vi "Set Temperature.vi"(8 "error in (no error)":errorcluster, 10 "Setpoint":dbl, 11 "HotCoil Settings":T1) -> (0 "error out":errorcluster, 1 "Connection Error":bool, 3 "HotCoil Settings":T1)   [LabVIEW 2021, in "HotCoil.lvlib"]
uses:
  HotCoil.lvlib
  HotCoil Settings.ctl
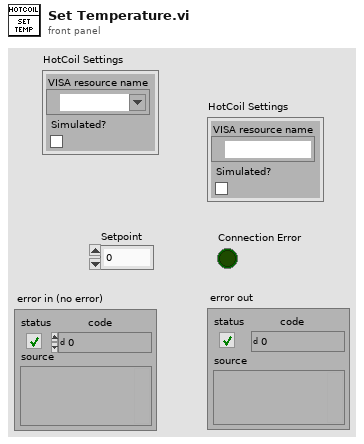
[diagram p1: front panel]
types:
  T1 = typedef "HotCoil.lvlib/HotCoil Settings.ctl" = cluster{"VISA resource name":refnum<visa-resource-name>, "Simulated?":bool}
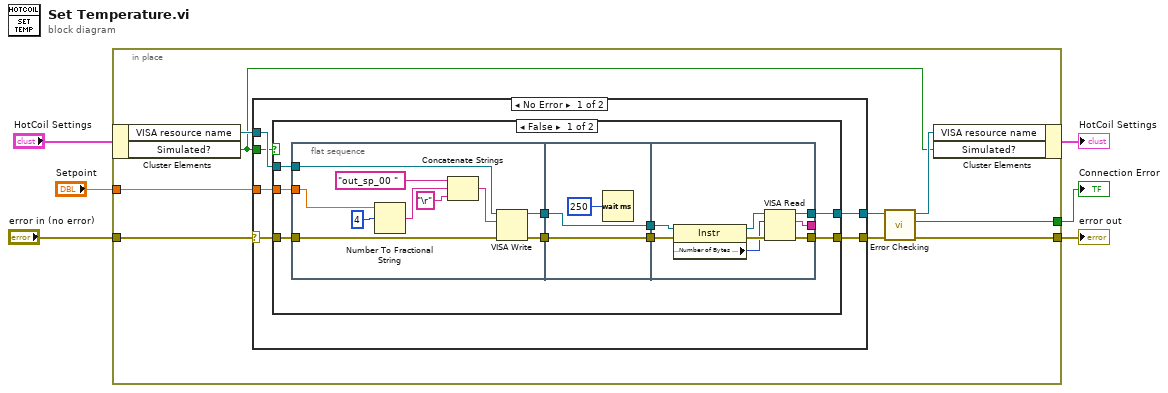
[diagram p0: block diagram]
diagram:
  n1 = in-place {
    in-place-border: "error in (no error)" -> [w15]
    in-place-border: [w12] -> w5
    in-place-border: [w11] -> w4
    in-place-border: "Setpoint" -> [w8]
    n2 = in-place-cluster #1("HotCoil Settings") -> ("VISA resource name"=w10:refnum<visa-resource-name>, "Simulated?"=w7:bool)
    n3 = case shown="No Error" w15 {
      selector: w15 -> [w21 w55]
      tunnel: [w20 w55] -> w13
      tunnel: [w19 w54] -> w14
      tunnel: w10 -> [w18 w54]
      tunnel: w8 -> [w17 _]
      tunnel: w7 -> [w16 _]
      frame No Error {
        n4 = case shown="False" w16 {
          tunnel: w21 -> [w25 w53]
          tunnel: [w23 w53] -> w20
          tunnel: [w24 w52] -> w19
          tunnel: w18 -> [w26 w52]
          tunnel: w17 -> [w22 _]
          frame False {
            n5 = flat-sequence {
              tunnel: w25 -> [w40]
              tunnel: w26 -> [w39]
              tunnel: [w38] -> w30
              tunnel: [w37] -> w29
              tunnel: w22 -> [w36]
              tunnel: w30 -> [w43]
              tunnel: [w43] -> w28
              tunnel: w29 -> [w42]
              tunnel: [w42] -> w27
              tunnel: [w51] -> w23
              tunnel: [w50] -> _
              tunnel: [w49] -> w24
              tunnel: w28 -> [w48]
              tunnel: w27 -> [w47]
              frame #0 {
                n6 = Number To Fractional String(number=w36, width (-)=i16 4) -> (F-format string=w33:string)  [unwired: 2 in]
                n7 = Concatenate Strings("out_sp_00 " ("write buffer"), w33, "\r" ("write buffer")) -> (w31:string)
                n8 = VISA Write(VISA resource name=w39, write buffer=w31, error in (no error)=w40) -> (VISA resource name out=w38:refnum<visa-resource-name>, error out=w37:errorcluster)  [unwired: 1 out]
              }
              frame #1 {
                n9 = Wait (ms)(milliseconds to wait=u32 250) -> ()  [unwired: 1 out]
              }
              frame #2 {
                n10 = property class="Instr"(reference=w48, error in=w47) -> (reference out=w46:refnum<visa-resource-name>, error out=w45:errorcluster, "Serial Settings:Number of Bytes at Serial Port"=w44:u32)
                n11 = VISA Read(VISA resource name=w46, byte count=w44, error in (no error)=w45) -> (VISA resource name out=w49:refnum<visa-resource-name>, read buffer=w50:string, error out=w51:errorcluster)  [unwired: 1 out]
              }
            }
          }
          frame True {
          }
        }
      }
      frame Error {
      }
    }
    n12 = call "Error Checking.vi"("error in (no error)"=w13, "VISA resource name"=w14) -> ("error out"=w12:errorcluster, "Connection Error"=w11:bool, "VISA resource name"=w9:refnum<visa-resource-name>)  [unwired: 7 in]
    n13 = in-place-cluster #1("VISA resource name"=w9, "Simulated?"=w7) -> (→"HotCoil Settings":T1)
  }
  "error out" <- w5
  "Connection Error" <- w4
